vi "Init Hardware.vi"(8 "error in (no error)":errorcluster, 11 "Ni-Scope Digitizer in":refnum<class "Ni-Scope Digitizer.lvclass">) -> (0 "error out":errorcluster, 3 "Ni-Scope Digitizer out":refnum<class "Ni-Scope Digitizer.lvclass">)   [LabVIEW 2016, in "Ni-Scope Digitizer.lvclass"]
uses:
  Ni-Scope Digitizer.lvclass
  C:/github/NHMFL_Core/Libraries/Instruments/Pulse Driver/Pulse Driver.lvclass
  <instrlib>/niScope/Controls/niScope trigger source digital.ctl
  Ni-Scope Digitizer.lvclass/Ni-Scope Digitizer.ctl
  Instruments/Pulse Driver/Pulse Driver.lvclass/Pulse Driver.ctl
  Read Device name.vi
  Instruments/Pulse Driver/Read Pretrigger samples.vi
  Instruments/Pulse Driver/Read Samples per channel.vi
  Read Triggering.vi
  Instruments/Pulse Driver/Write Samples per channel.vi
  Instruments/Pulse Driver/Write dt.vi
  Instruments/Pulse Driver/Write t0.vi
  Instruments/Pulse Driver/Write Set timing from UI.vi
  Instruments/Pulse Driver/Write Binary sample width.vi
  Write instrument handle.vi
  <instrlib>/niScope/Configure/Trigger/niScope Configure Trigger Software.vi
  <instrlib>/niScope/Configure/Trigger/niScope Configure Trigger Digital.vi
  <instrlib>/niScope/Acquire/niScope Get Scaling Coefficients.vi
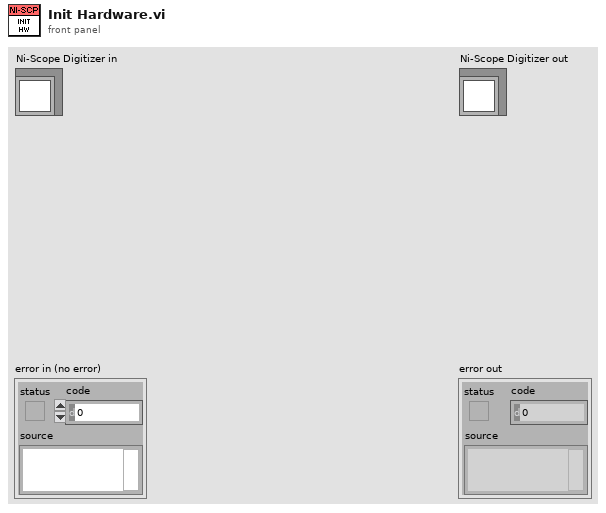
[diagram p1: front panel]
types:
  T1 = typedef "niScope trigger source digital.ctl" = string
  T2 = typedef "Pusle Driver Configuration.ctl" = cluster{"Pre-trigger duration":dbl, "Post-trigger duration":dbl, "Rate":dbl, "Ranges":dbl[], "Re-name channels":string[], "Active channels":string, "External clock":bool}
  T3 = cluster{"offset":dbl, "gain":dbl, "reserved 1":dbl, "reserved 2":dbl}[]
  T4 = cluster{"offset":dbl, "gain":dbl, "reserved 1":dbl, "reserved 2":dbl}
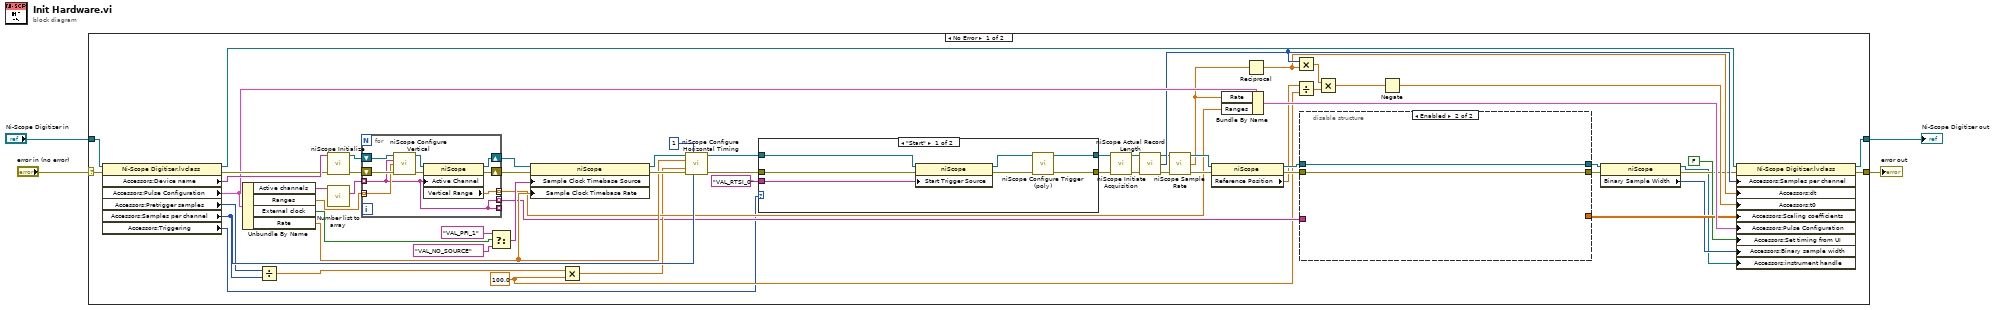
[diagram p0: block diagram]
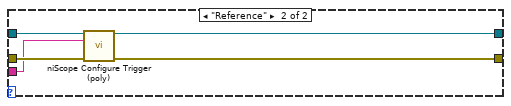
[diagram p2: hidden frame]
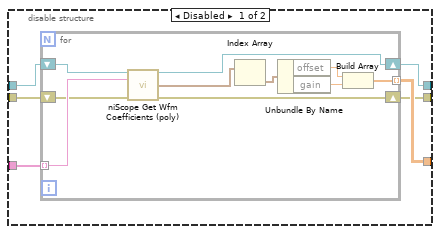
[diagram p3: hidden frame]
diagram:
  n1 = case shown="No Error" "error in (no error)" {
    selector: "error in (no error)" -> [w55 w105]
    tunnel: [w27 w105] -> w3
    tunnel: [w28 w104] -> w1
    tunnel: "Ni-Scope Digitizer in" -> [w34 w104]
    frame No Error {
      w16 = 100.0 ("y")
      n2 = property class="Ni-Scope Digitizer.lvclass"(reference=w34, error in=w55) -> (reference out=w29:refnum<class "Ni-Scope Digitizer.lvclass">, error out=w56:errorcluster, "Accessors:Device name"=w57:string, "Accessors:Pulse Configuration"=w43:T2, "Accessors:Pretrigger samples"=w53:u32, "Accessors:Samples per channel"=w54:i32, "Accessors:Triggering"=w10:enum16{"Reference", "Start"})
      n3 = Unbundle By Name(w43) -> ("Active channels"=w60:string, "Ranges"=w58:dbl[], "External clock"=w48:bool, "Rate"=w44:dbl)
      n4 = Divide(x=w53, y=w54) -> (x/y=w61:dbl)
      n5 = call <instrlib>:"niScope Initialize.vi"("resource name"=w57, "error in"=w56) -> ("instrument handle"=w63:refnum<k15>, "error out"=w64:errorcluster)  [unwired: 2 in, 10 out]
      n6 = call "Number list to array.vi"("Number list"=w60) -> ("Full names"=w59:string[])  [unwired: 9 in, 1 out]
      n7 = for {
        tunnel: w58 -> [w101] mode=indexing
        shift-right: [w97] -> w51
        shift-left: w64 -> [w103]
        shift-right: [w99] -> w52
        shift-left: w63 -> [w102]
        tunnel: w59 -> [w95] mode=indexing
        tunnel: [w95] -> _ mode=indexing
        tunnel: [w96] -> w33 mode=indexing
        tunnel: [w95] -> w31 mode=indexing
        n8 = call <instrlib>:"niScope Configure Vertical.vi"("instrument handle"=w102, "channels"=w95, "vertical range"=w101, "error in"=w103) -> ("instrument handle out"=w100:refnum<k15>, "error out"=w98:errorcluster)  [unwired: 10 in]
        n9 = property class="niScope"(reference=w100, error in=w98, "Active Channel"=w95) -> (reference out=w99:refnum<k15>, error out=w97:errorcluster, "Vertical Range"=w96:dbl)
      }
      n10 = Select(t="VAL_PFI_1", s=w48, f="VAL_NO_SOURCE") -> (s? t:f=w45:string)
      n11 = property class="niScope"(reference=w52, error in=w51, "Sample Clock Timebase Source"=w45, "Sample Clock Timebase Rate"=w44) -> (reference out=w50:refnum<k15>, error out=w49:errorcluster)
      n12 = Multiply(x=w61, y=w16) -> (x*y=w32:dbl)
      n13 = call <instrlib>:"niScope Configure Horizontal Timing.vi"("instrument handle"=w50, "number of records"=1, "min sample rate"=w44, "reference position"=w32, "error in"=w49, "min record length"=w54) -> ("instrument handle out"=w9:refnum<k15>, "error out"=w7:errorcluster)  [unwired: 1 in, 7 out]
      n14 = case shown="\"Start\"" w10 {
        tunnel: w9 -> [w71 w76]
        tunnel: w7 -> [w66 w75]
        tunnel: T1 "VAL_RTSI_0" ("trigger source") -> [w65 w74]
        tunnel: [w70 w73] -> w6
        tunnel: [w69 w72] -> w5
        frame "Start" {
          n15 = property class="niScope"(reference=w71, error in=w66, "Start Trigger Source"=w65) -> (reference out=w68:refnum<k15>, error out=w67:errorcluster)
          n16 = call-poly <instrlib>:"niScope Configure Trigger (poly).vi"("instrument handle"=w68, "error in"=w67) -> ("instrument handle out"=w70:refnum<k15>, "error out"=w69:errorcluster)  [unwired: 12 in]
        }
        frame "Reference" {
          n17 = call-poly <instrlib>:"niScope Configure Trigger (poly).vi"("instrument handle"=w76, "trigger source"=w74, "error in"=w75) -> ("instrument handle out"=w73:refnum<k15>, "error out"=w72:errorcluster)  [unwired: 11 in]
        }
      }
      n18 = call <instrlib>:"niScope Initiate Acquisition.vi"("instrument handle"=w6, "error in"=w5) -> ("instrument handle out"=w26:refnum<k15>, "error out"=w23:errorcluster)  [unwired: 12 in]
      n19 = call <instrlib>:"niScope Actual Record Length.vi"("instrument handle"=w26, "error in"=w23) -> ("instrument handle out"=w25:refnum<k15>, "actual record length"=w39:i32, "error out"=w24:errorcluster)  [unwired: 11 out]
      n20 = call <instrlib>:"niScope Sample Rate.vi"("instrument handle"=w25, "error in"=w24) -> ("instrument handle out"=w42:refnum<k15>, "actual sample rate"=w30:dbl, "error out"=w41:errorcluster)  [unwired: 11 out]
      n21 = property class="niScope"(reference=w42, error in=w41) -> (reference out=w22:refnum<k15>, error out=w21:errorcluster, "Reference Position"=w17:dbl)
      n22 = Bundle By Name(cluster=w43, "Rate"=w30, "Ranges"=w33) -> (w40:T2)
      n23 = Reciprocal(x=w30) -> (1/x=w38:dbl)
      n24 = Multiply(x=w39, y=w38) -> (x*y=w37:dbl)
      n25 = Divide(x=w17, y=w16) -> (x/y=w18:dbl)
      n26 = disable-structure shown="Enabled" {
        disable-tunnel: w31 -> [w82 _]
        disable-tunnel: w22 -> [w81 w93]
        disable-tunnel: w21 -> [w80 w94]
        disable-tunnel: [w79 _] -> w20
        disable-tunnel: [w78 w93] -> w15
        disable-tunnel: [w77 w94] -> w14
        frame Disabled {
          n27 = for {
            tunnel: w82 -> [w84] mode=indexing
            shift-right: [w91] -> w77
            shift-left: w80 -> [w83]
            shift-right: [w92] -> w78
            shift-left: w81 -> [w85]
            tunnel: [w86] -> w79 mode=indexing
            n28 = call-poly <instrlib>:"niScope Get Wfm Coefficients (poly).vi"("instrument handle"=w85, "channels"=w84, "error in"=w83) -> ("instrument handle out"=w92:refnum<k15>, "coefficient info"=w90:T3, "error out"=w91:errorcluster)  [unwired: 10 in]
            n29 = Index Array(array=w90) -> (element=w89:T4)  [unwired: 1 in]
            n30 = Unbundle By Name(w89) -> ("offset"=w88:dbl, "gain"=w87:dbl)
            n31 = Build Array(w88, w87) -> (w86:dbl[])
          }
        }
        frame Enabled {
        }
      }
      n32 = Multiply(x=w37, y=w18) -> (x*y=w36:dbl)
      n33 = Negate(x=w36) -> (-x=w35:dbl)
      n34 = property class="niScope"(reference=w15, error in=w14) -> (reference out=w11:refnum<k15>, error out=w13:errorcluster, "Binary Sample Width"=w12:i32)
      n35 = property class="Ni-Scope Digitizer.lvclass"(reference=w29, error in=w13, "Accessors:Samples per channel"=w39, "Accessors:dt"=w38, "Accessors:t0"=w35, "Accessors:Scaling coefficients"=w20, "Accessors:Pulse Configuration"=w40, "Accessors:Set timing from UI"=FALSE ("Set timing from UI"), "Accessors:Binary sample width"=w12, "Accessors:instrument handle"=w11) -> (reference out=w28:refnum<class "Ni-Scope Digitizer.lvclass">, error out=w27:errorcluster)
    }
    frame Error {
    }
  }
  "error out" <- w3
  "Ni-Scope Digitizer out" <- w1
